vi "Clappy up down.vi"(0 "Manual":bool, 1 "Open/Closed 1":dbl, 2 "Open/Closed 2":dbl, 3 "UP/Down":dbl, 7 "Negate 1":bool, 9 "Negate 2":bool) -> ()   [LabVIEW 2015]
uses:
  <vilib>/Rock Robotics/WPI/Utilities/WPI_GetSetVariantRefNum.vi
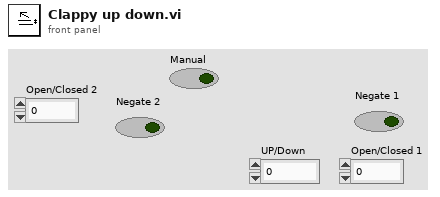
[diagram p1: front panel]
types:
  T1 = typedef "WPI_RobotDriveDevRef.ctl" = cluster{"DevStatus":errorcluster, "Motors[]":T2[], "Square Inputs":bool, "Max Output":dbl}
  T2 = typedef "WPI_MotorControlDeviceRef.ctl" = cluster{"DeviceStatus":errorcluster, "Type":T3, "PWM":cluster{"PWM Channel":T4, "DeadBand":T5}, "CAN":cluster{"Device Number":u8, "Control Mode":T6, "Semaphore":T7, "Max Vout":dbl, "TalonSRX Control Mode":T8}, "Invert":bool}
  T3 = typedef "WPI_MotorControlType.ctl" = enum16{"PWM", "CAN", "CANTalonSRX"}
  T4 = typedef "FPGA_DIOPWMChannel.ctl" = enum8{"PWM 0", "PWM 1", "PWM 2", "PWM 3", "PWM 4", "PWM 5", "PWM 6", "PWM 7", "PWM 8", "PWM 9", "PWM MXP 0", "PWM MXP 1", "PWM MXP 2", "PWM MXP 3", "PWM MXP 4", "PWM MXP 5", "PWM MXP 6", "PWM MXP 7", "PWM MXP 8", "PWM MXP 9", "Invalid"}
  T5 = typedef "WPI_PWMDeadband.ctl" = cluster{"Name":string, "maxPositivePwm":i32, "minPositivePwm":i32, "centerPwm":i32, "maxNegativePwm":i32, "minNegativePwm":i32, "angularRange":u16}
  T6 = typedef "WPI_CANJaguar_ControlMode.ctl" = enum8{"Percent VBus", "Current", "Speed", "Position", "Voltage"}
  T7 = typedef "Semaphore RefNum" = refnum<k1>
  T8 = typedef "WPI_CANTalonSRX_APIControlMode.ctl" = enum8{"Percent VBus", "Speed", "Position", "Slave", "Unchanged / Invalid", "Voltage Compensation", "Current", "Motion Profile"}
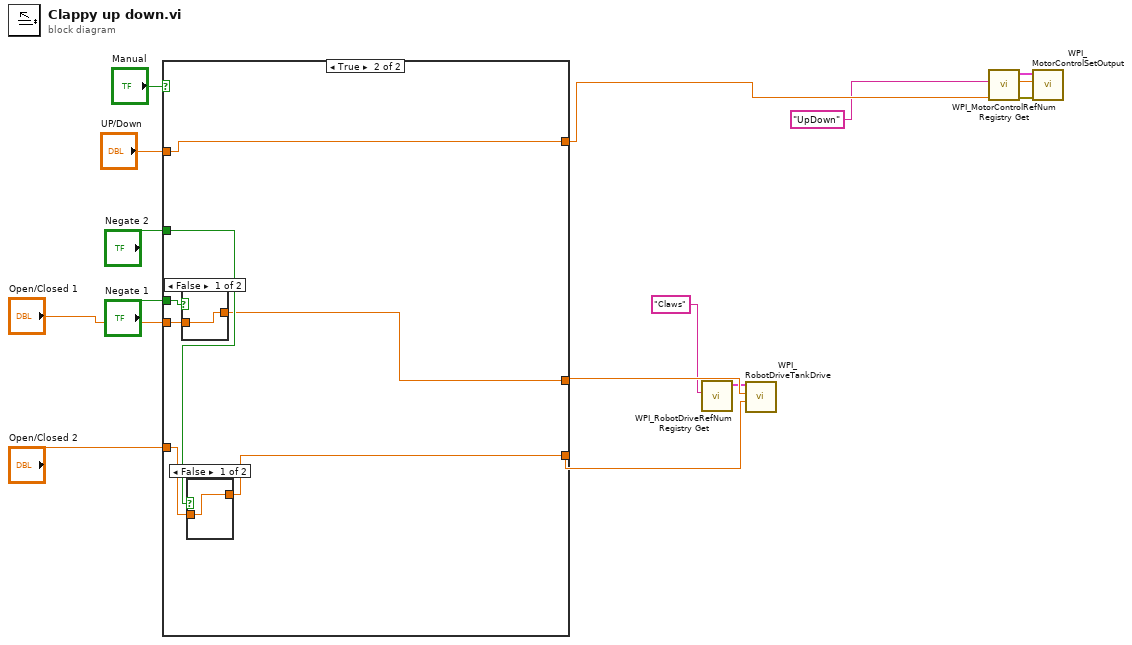
[diagram p0: block diagram]
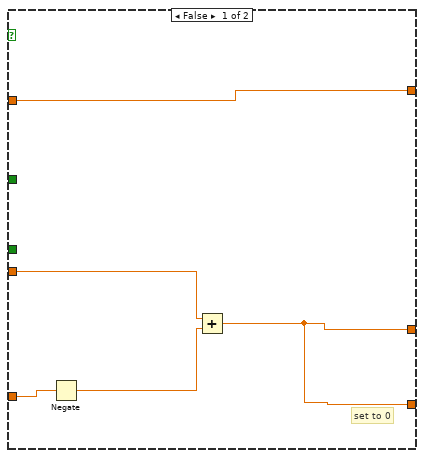
[diagram p2: hidden frame]
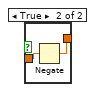
[diagram p3: hidden frame]
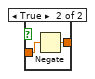
[diagram p4: hidden frame]
diagram:
  n1 = case shown="True" "Manual" {
    tunnel: "Open/Closed 1" -> [w17 w24]
    tunnel: "UP/Down" -> [w15 w20]
    tunnel: "Negate 1" -> [_ w26]
    tunnel: [w15 w20] -> w6
    tunnel: [w16 w22] -> w9
    tunnel: [w16 w21] -> w10
    tunnel: "Negate 2" -> [_ w25]
    tunnel: "Open/Closed 2" -> [w19 w23]
    frame False {
      # "set to 0"
      n2 = Negate(x=w19) -> (-x=w18:dbl)
      n3 = Add(x=w17, y=w18) -> (x+y=w16:dbl)
    }
    frame True {
      n4 = case shown="False" w26 {
        tunnel: w24 -> [w30 w32]
        tunnel: [w30 w31] -> w21
        frame False {
        }
        frame True {
          n5 = Negate(x=w32) -> (-x=w31:dbl)
        }
      }
      n6 = case shown="False" w25 {
        tunnel: w23 -> [w27 w29]
        tunnel: [w27 w28] -> w22
        frame False {
        }
        frame True {
          n7 = Negate(x=w29) -> (-x=w28:dbl)
        }
      }
    }
  }
  n8 = call <vilib>:"WPI_RobotDriveRefNum Registry Get.vi"("refnum name"="Claws") -> ("RobotDriveDevRef"=w4:T1)  [unwired: 9 in, 1 out]
  n9 = call <vilib>:"WPI_RobotDriveTankDrive.vi"("Right axis value"=w9, "Left axis value"=w10, "RobotDriveDevRef"=w4) -> ()  [unwired: 6 in, 3 out]
  n10 = call <vilib>:"WPI_MotorControlRefNum Registry Get.vi"("refnum name"="UpDown") -> ("error out"=w3:errorcluster, "MotorControlDevRef"=w2:T2)  [unwired: 9 in]
  n11 = call <vilib>:"WPI_MotorControlSetOutput.vi"("error in (no error)"=w3, "Output"=w6, "MotorControlDevRef"=w2) -> ()  [unwired: 6 in, 3 out]
